vi "ListDependencies.vi"(8 "error in (no error)":errorcluster, 11 "SMO in":refnum<class "SMO.lvclass">) -> (0 "error out":errorcluster, 1 "Level":string[](array[string]), 2 "[Dependencies]":refnum<class "SMO.lvclass">[](array[class]), 3 "SMO out":refnum<class "SMO.lvclass">)   [LabVIEW 2021, in "smo.lvlib" / "SMO.lvclass"]
uses:
  SMO.lvclass
  SMO.lvclass/SMO.ctl
  Private/GetVariant(Attr).vi
  Private/ReftoDVR--SMO.vi
  Support/Attribute.Dependencies/Get GUIDs.vi
  Support/Attribute.Dependencies/Attribute.Dependencies.lvclass
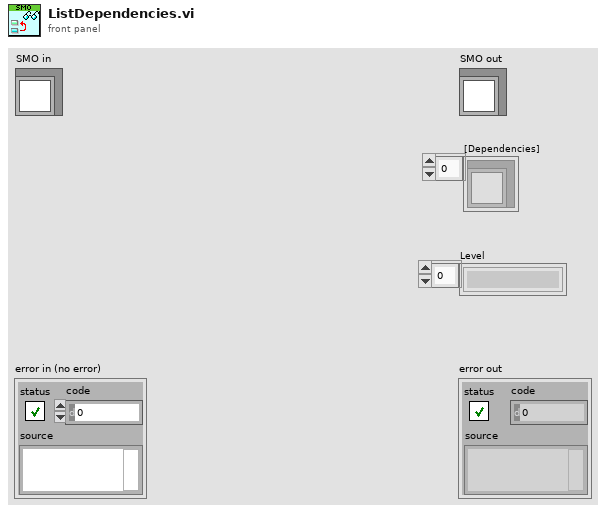
[diagram p1: front panel]
types:
  T1 = typedef "smo.lvlib/Attribute.Dependencies.lvclass/DependencyAttr--Cluster.ctl" = cluster{"Name":string, "GUID":string, "owned":bool, "shared":bool, "Level":string, "SMO":refnum<class "SMO.lvclass">}
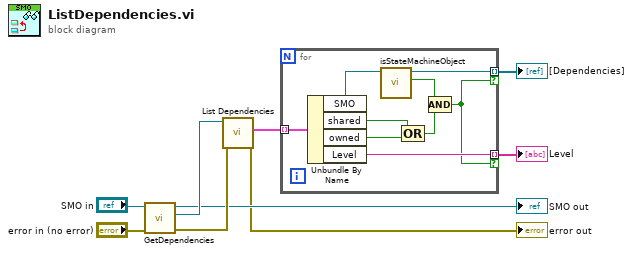
[diagram p0: block diagram]
diagram:
  n1 = call "GetDependencies.vi"("error in (no error)"="error in (no error)", "SMO in"="SMO in") -> ("error out"=w3:errorcluster, "Dependencies"=w6:refnum<class "Attribute.Dependencies.lvclass">, "SMO out"=→"SMO out":refnum<class "SMO.lvclass">)  [unwired: 7 in]
  n2 = call "List Dependencies.vi"("error in (no error)"=w3, "Attribute.Dependencies in"=w6) -> ("error out"=→"error out":errorcluster, "Dependencies"=w5:T1[])  [unwired: 7 in, 1 out]
  n3 = for {
    tunnel: [w14] -> w9 mode=indexing if=w11
    tunnel: [w17] -> w8 mode=indexing if=w11
    tunnel: w5 -> [w18] mode=indexing
    n4 = Unbundle By Name(w18) -> ("SMO"=w15:refnum<class "SMO.lvclass">, "shared"=w16:bool, "owned"=w13:bool, "Level"=w17:string)
    n5 = call "isStateMachineObject.vi"("SMO"=w15) -> ("is SMO?"=w10:bool, "SMO out"=w14:refnum<class "SMO.lvclass">)  [unwired: 8 in, 1 out]
    n6 = Compound Arithmetic op=OR(w16, w13) -> (w12:bool)
    n7 = Compound Arithmetic op=AND(w10, w12) -> (w11:bool)
  }
  "[Dependencies]" <- w9
  "Level" <- w8
